vi "Create Process.vi"(8 "error in (no error)":errorcluster, 10 "Sequence":string[](array[string]), 11 "Process Model in":refnum<class "Process Model.lvclass">) -> (0 "error out":errorcluster, 3 "Process Model out":refnum<class "Process Model.lvclass">)   [LabVIEW 2017, in "Process Model.lvlib" / "Process Model.lvclass"]
uses:
  <vilib>/gpm_packages/@cs/Car wash/Process Model/Process Model/Process Model.lvclass
  <vilib>/gpm_packages/@cs/test-executive/Source/Test Executive/TestExecutive Ref/TestExecutive Ref.lvclass
  <vilib>/gpm_packages/@cs/test-executive/Source/Test Executive/TestExecutive/Test Executive.lvclass
  <vilib>/gpm_packages/@cs/Car wash/Process Model/Process Steps/Set Desired Station/Set Desired Station.lvclass
  <vilib>/gpm_packages/@cs/test-executive/Source/Test Executive/Executioner/Executioner.lvclass
  148baa78-ab47-4ac2-a908-5eab3e623dd9.vi
  2634eeb6-4d42-4bc9-82b5-37b6fa3864e8.vi
  <vilib>/gpm_packages/@cs/Car wash/Process Model/Process Steps/Start Under Body Wash/Start Under Body Wash.lvclass
  e4c6561f-6417-4e21-a938-d836dda1ae79.vi
  <vilib>/gpm_packages/@cs/Car wash/Process Model/Process Steps/Wait/Wait.lvclass
  c08b7c41-2827-4655-bbff-50a6a7c73d4f.vi
  <vilib>/gpm_packages/@cs/Car wash/Process Model/Process Steps/Stop Under Body Wash/Stop Under Body Wash.lvclass
  f4110d32-f2ed-440d-ac33-f75860a216d9.vi
  <vilib>/gpm_packages/@cs/Car wash/Process Model/Process Steps/Start Bug Remover/Start Bug Remover.lvclass
  38c94591-f339-49dc-907e-f278cc2e51ff.vi
  <vilib>/gpm_packages/@cs/Car wash/Process Model/Process Steps/Stop Bug Remover/Stop Bug Remover.lvclass
  f7fd6c87-c4ae-48d3-978c-34364638cacd.vi
  <vilib>/gpm_packages/@cs/Car wash/Process Model/Process Steps/Start Pre-Soak/Start Pre-Soak.lvclass
  975d0a21-73d7-4169-b5a5-a1460635b443.vi
  <vilib>/gpm_packages/@cs/Car wash/Process Model/Process Steps/Stop Pre-Soak/Stop Pre-Soak.lvclass
  07d419d3-c35c-4609-8eee-0d116beaf2ef.vi
  <vilib>/gpm_packages/@cs/Car wash/Process Model/Process Steps/Start High Pressure Wash/Start High Pressure Wash.lvclass
  43e1845e-1a9b-47c3-a4cd-faa5e21737b1.vi
  <vilib>/gpm_packages/@cs/Car wash/Process Model/Process Steps/Stop High Pressure Wash/Stop High Pressure Wash.lvclass
  178d77fd-57ed-4720-a89c-829f4238c359.vi
  <vilib>/gpm_packages/@cs/Car wash/Process Model/Process Steps/Start Low Pressure Wax/Start Low Pressure Wax.lvclass
  1292d9c1-c930-4c00-a311-9cd2a177a2f0.vi
  <vilib>/gpm_packages/@cs/Car wash/Process Model/Process Steps/Stop Low Pressure Wax/Stop Low Pressure Wax.lvclass
  f597536c-d9cd-43c5-8d13-b9a318907401.vi
  <vilib>/gpm_packages/@cs/Car wash/Process Model/Process Steps/Start Air Dry/Start Air Dry.lvclass
  adc60016-b060-4db0-b707-518d8c9f6844.vi
  <vilib>/gpm_packages/@cs/Car wash/Process Model/Process Steps/Stop Air Dry/Stop Air Dry.lvclass
  58db1882-6cd1-40bb-add2-e4b922ecf0a5.vi
  <vilib>/gpm_packages/@cs/Car wash/Process Model/Process Steps/Start Spot Free Rinse/Start Spot Free Rinse.lvclass
  7577cb98-fec7-4599-9fc4-8f1fe5d712e2.vi
  <vilib>/gpm_packages/@cs/Car wash/Process Model/Process Steps/Stop Spot Free Rinse/Stop Spot Free Rinse.lvclass
  fc6307b7-2fc7-402e-94d3-f9c0f8fc91bb.vi
  <vilib>/gpm_packages/@cs/Car wash/Process Model/Process Steps/Start Tire Shine Foam/Start Tire Shine Foam.lvclass
  13563156-251b-405d-92c3-91e0f6b0e34d.vi
  <vilib>/gpm_packages/@cs/Car wash/Process Model/Process Steps/Stop Tire Shine Foam/Stop Tire Shine Foam.lvclass
  640e79f8-33ad-472c-aa49-3045e868de91.vi
  <vilib>/gpm_packages/@cs/Car wash/Process Model/Process Steps/Exit/Exit.lvclass
  b05cf328-ca6c-4f2d-8483-90633d7417f2.vi
  <vilib>/gpm_packages/@cs/Car wash/Process Model/Process Steps/Initialize HMI/Initialize HMI.lvclass
  C:/Program Files/National Instruments/LabVIEW 2017/vi.lib/gpm_packages/@cs/test-executive/Source/Test Executive/ITestExecutive/ITest Executive.lvclass
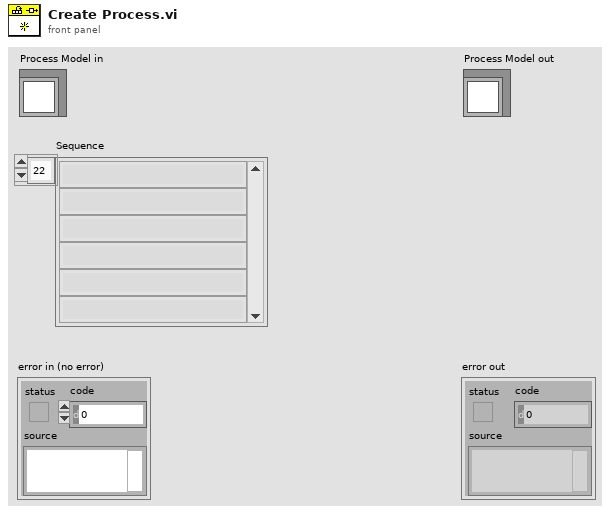
[diagram p1: front panel]
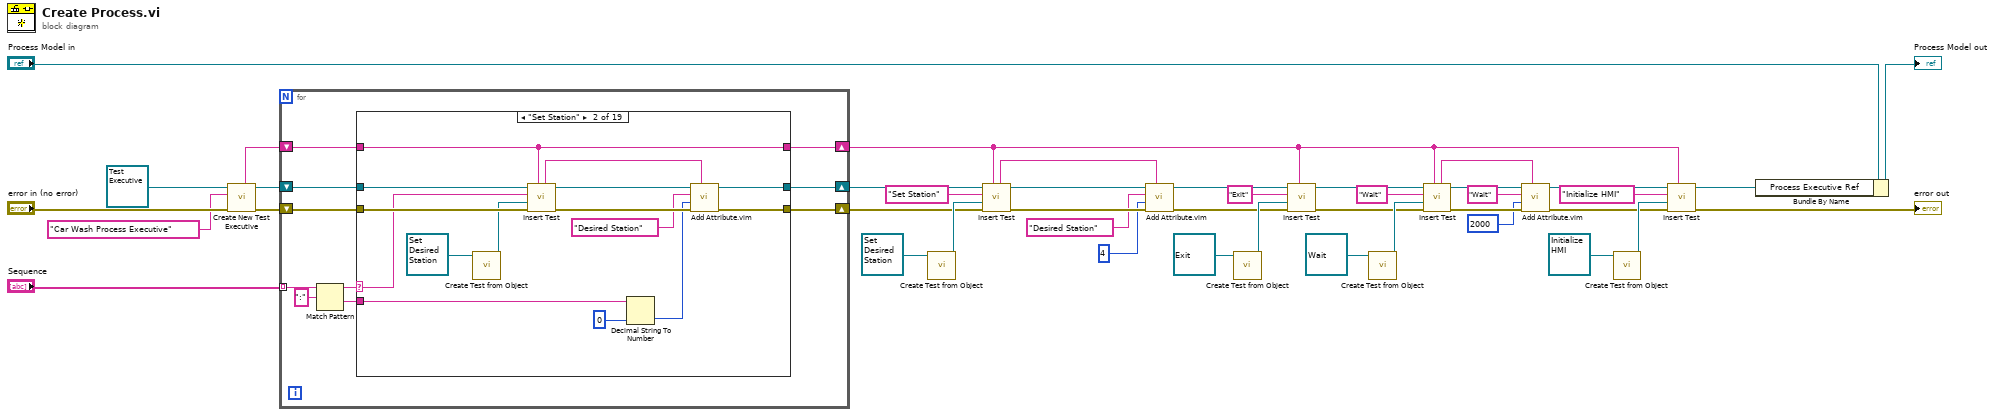
[diagram p0: block diagram]
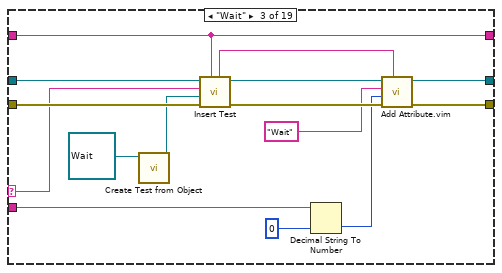
[diagram p3: hidden frame]
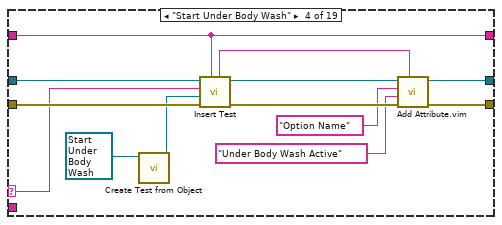
[diagram p4: hidden frame]
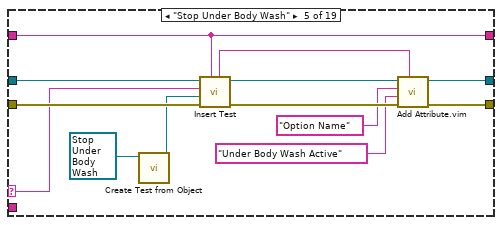
[diagram p5: hidden frame]
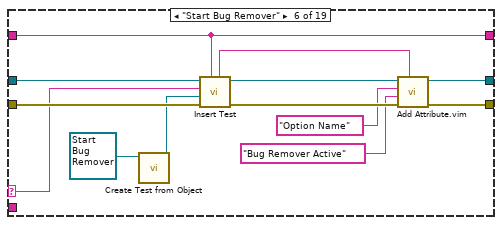
[diagram p6: hidden frame]
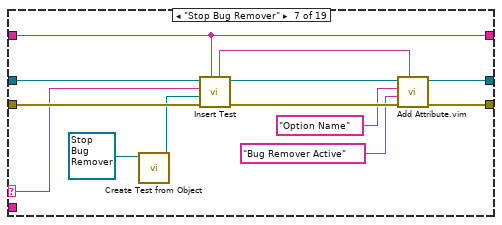
[diagram p7: hidden frame]
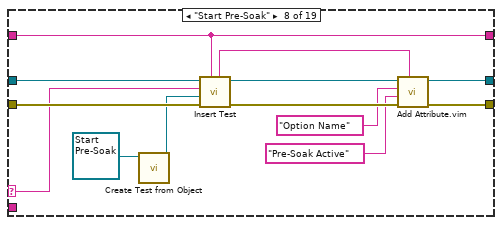
[diagram p8: hidden frame]
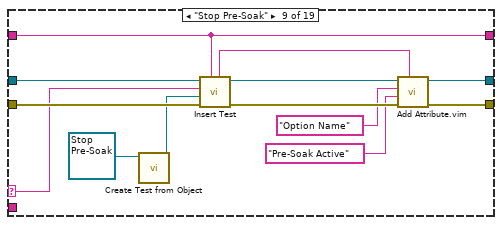
[diagram p9: hidden frame]
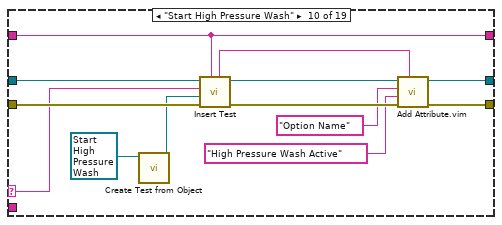
[diagram p10: hidden frame]
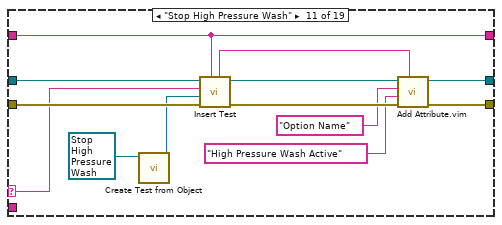
[diagram p11: hidden frame]
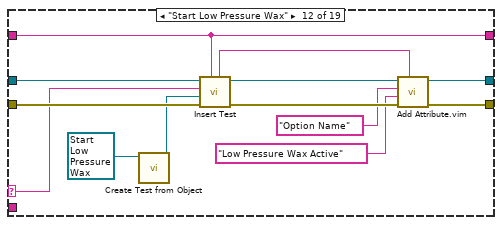
[diagram p12: hidden frame]
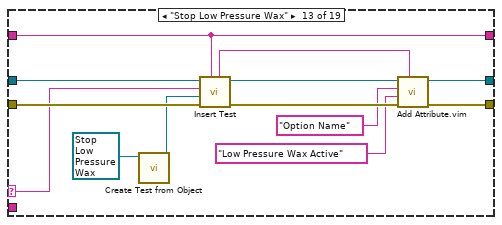
[diagram p13: hidden frame]
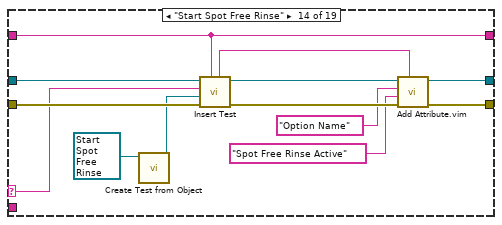
[diagram p14: hidden frame]
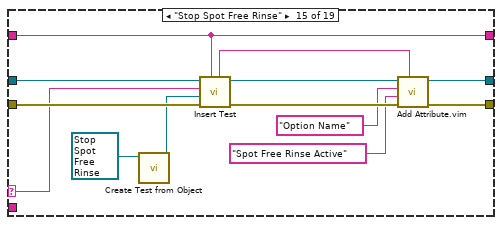
[diagram p15: hidden frame]
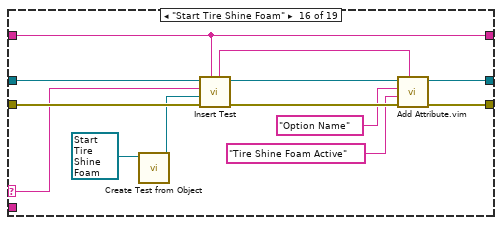
[diagram p16: hidden frame]
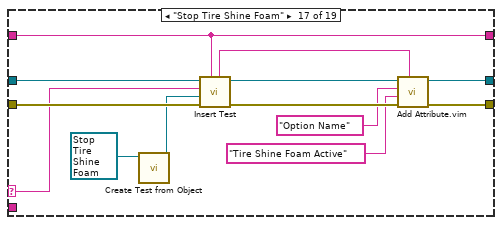
[diagram p17: hidden frame]
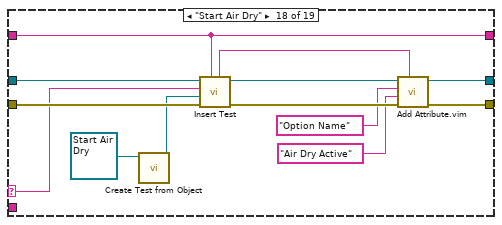
[diagram p18: hidden frame]
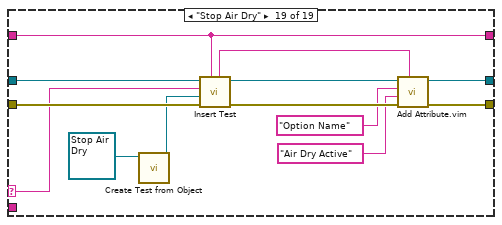
[diagram p19: hidden frame]
diagram:
  n1 = call <vilib>:"Create New Test Executive.vi"("error in (no error)"="error in (no error)", "Name"="Car Wash Process Executive", "Test Executive"=refnum<class "Test Executive.lvclass"> refnum ("Test Executive.lvlib:Test Executive.lvclass")) -> ("error out"=w36:errorcluster, "Test Executive Ref"=w37:refnum<data-value>, "Test Executive ID out"=w34:string)  [unwired: 6 in]
  n2 = for {
    shift-right: [w51] -> w27
    shift-left: w37 -> [w52]
    shift-right: [w49] -> w26
    shift-left: w36 -> [w50]
    tunnel: "Sequence" -> [w48] mode=indexing
    shift-right: [w43] -> w4
    shift-left: w34 -> [w44]
    n3 = Match Pattern(string=w48, regular expression=":") -> (before substring=w47:string, after substring=w46:string)  [unwired: 1 in, 2 out]
    n4 = case shown="\"Set Station\"" w47 {
      selector: w47 -> [_ w68 w82 w95 w108 w121 w134 w147 w160 w173 w186 w199 w212 w225 w238 w251 w264 w277 w290]
      tunnel: w52 -> [w55 w70 w85 w98 w111 w124 w137 w150 w163 w176 w189 w202 w215 w228 w241 w254 w267 w280 w293]
      tunnel: [w55 w64 w79 w92 w105 w118 w131 w144 w157 w170 w183 w196 w209 w222 w235 w248 w261 w274 w287] -> w51
      tunnel: w50 -> [w54 w69 w84 w97 w110 w123 w136 w149 w162 w175 w188 w201 w214 w227 w240 w253 w266 w279 w292]
      tunnel: [w54 w62 w77 w90 w103 w116 w129 w142 w155 w168 w181 w194 w207 w220 w233 w246 w259 w272 w285] -> w49
      tunnel: w46 -> [_ w59 w75 _ _ _ _ _ _ _ _ _ _ _ _ _ _ _ _]
      tunnel: w44 -> [w53 w56 w83 w96 w109 w122 w135 w148 w161 w174 w187 w200 w213 w226 w239 w252 w265 w278 w291]
      tunnel: [w53 w56 w83 w96 w109 w122 w135 w148 w161 w174 w187 w200 w213 w226 w239 w252 w265 w278 w291] -> w43
      frame Default {
      }
      frame "Set Station" {
        n5 = call <vilib>:"Create Test from Object.vi"("Test"=refnum<class "Set Desired Station.lvclass"> refnum ("Set Desired Station.lvclass")) -> ("Test"=w66:refnum<class "Executioner.lvclass">)  [unwired: 10 in]
        n6 = call <vilib>:"Insert Test.vi"("Parent ID"=w56, "error in (no error)"=w69, "Test"=w66, "Name"=w68, "Test Executive Ref"=w70) -> ("error out"=w63:errorcluster, "Test Executive Ref out"=w65:refnum<data-value>, "Unique ID out"=w61:string)  [unwired: 3 in, 1 out]
        n7 = Decimal String To Number(string=w59, default (0L)=u8 0) -> (number=w57:u8)  [unwired: 1 in, 1 out]
        n8 = call "Add Attribute.vim"("ID"=w61, "error in (no error)"=w63, "Attribute"=w57, "Attribute Name"="Desired Station" ("Item Name"), "Test Executive Ref"=w65) -> ("error out"=w62:errorcluster, "Test Executive Ref out"=w64:refnum<data-value>)  [unwired: 3 in, 2 out]
      }
      frame "Wait" {
        n9 = call <vilib>:"Create Test from Object.vi"("Test"=refnum<class "Wait.lvclass"> refnum ("Wait.lvclass")) -> ("Test"=w81:refnum<class "Executioner.lvclass">)  [unwired: 10 in]
        n10 = call <vilib>:"Insert Test.vi"("Parent ID"=w83, "error in (no error)"=w84, "Test"=w81, "Name"=w82, "Test Executive Ref"=w85) -> ("error out"=w78:errorcluster, "Test Executive Ref out"=w80:refnum<data-value>, "Unique ID out"=w76:string)  [unwired: 3 in, 1 out]
        n11 = Decimal String To Number(string=w75, default (0L)=0) -> (number=w74:i32)  [unwired: 1 in, 1 out]
        n12 = call "Add Attribute.vim"("ID"=w76, "error in (no error)"=w78, "Attribute"=w74, "Attribute Name"="Wait" ("Item Name"), "Test Executive Ref"=w80) -> ("error out"=w77:errorcluster, "Test Executive Ref out"=w79:refnum<data-value>)  [unwired: 3 in, 2 out]
      }
      frame "Start Under Body Wash" {
        n13 = call <vilib>:"Create Test from Object.vi"("Test"=refnum<class "Start Under Body Wash.lvclass"> refnum ("Start Under Body Wash.lvclass")) -> ("Test"=w94:refnum<class "Executioner.lvclass">)  [unwired: 10 in]
        n14 = call <vilib>:"Insert Test.vi"("Parent ID"=w96, "error in (no error)"=w97, "Test"=w94, "Name"=w95, "Test Executive Ref"=w98) -> ("error out"=w91:errorcluster, "Test Executive Ref out"=w93:refnum<data-value>, "Unique ID out"=w89:string)  [unwired: 3 in, 1 out]
        n15 = call "Add Attribute.vim"("ID"=w89, "error in (no error)"=w91, "Attribute"="Under Body Wash Active" ("Item Name"), "Attribute Name"="Option Name" ("Item Name"), "Test Executive Ref"=w93) -> ("error out"=w90:errorcluster, "Test Executive Ref out"=w92:refnum<data-value>)  [unwired: 3 in, 2 out]
      }
      frame "Stop Under Body Wash" {
        n16 = call <vilib>:"Create Test from Object.vi"("Test"=refnum<class "Stop Under Body Wash.lvclass"> refnum ("Stop Under Body Wash.lvclass")) -> ("Test"=w107:refnum<class "Executioner.lvclass">)  [unwired: 10 in]
        n17 = call <vilib>:"Insert Test.vi"("Parent ID"=w109, "error in (no error)"=w110, "Test"=w107, "Name"=w108, "Test Executive Ref"=w111) -> ("error out"=w104:errorcluster, "Test Executive Ref out"=w106:refnum<data-value>, "Unique ID out"=w102:string)  [unwired: 3 in, 1 out]
        n18 = call "Add Attribute.vim"("ID"=w102, "error in (no error)"=w104, "Attribute"="Under Body Wash Active" ("Item Name"), "Attribute Name"="Option Name" ("Item Name"), "Test Executive Ref"=w106) -> ("error out"=w103:errorcluster, "Test Executive Ref out"=w105:refnum<data-value>)  [unwired: 3 in, 2 out]
      }
      frame "Start Bug Remover" {
        n19 = call <vilib>:"Create Test from Object.vi"("Test"=refnum<class "Start Bug Remover.lvclass"> refnum ("Start Bug Remover.lvclass")) -> ("Test"=w120:refnum<class "Executioner.lvclass">)  [unwired: 10 in]
        n20 = call <vilib>:"Insert Test.vi"("Parent ID"=w122, "error in (no error)"=w123, "Test"=w120, "Name"=w121, "Test Executive Ref"=w124) -> ("error out"=w117:errorcluster, "Test Executive Ref out"=w119:refnum<data-value>, "Unique ID out"=w115:string)  [unwired: 3 in, 1 out]
        n21 = call "Add Attribute.vim"("ID"=w115, "error in (no error)"=w117, "Attribute"="Bug Remover Active" ("Item Name"), "Attribute Name"="Option Name" ("Item Name"), "Test Executive Ref"=w119) -> ("error out"=w116:errorcluster, "Test Executive Ref out"=w118:refnum<data-value>)  [unwired: 3 in, 2 out]
      }
      frame "Stop Bug Remover" {
        n22 = call <vilib>:"Create Test from Object.vi"("Test"=refnum<class "Stop Bug Remover.lvclass"> refnum ("Stop Bug Remover.lvclass")) -> ("Test"=w133:refnum<class "Executioner.lvclass">)  [unwired: 10 in]
        n23 = call <vilib>:"Insert Test.vi"("Parent ID"=w135, "error in (no error)"=w136, "Test"=w133, "Name"=w134, "Test Executive Ref"=w137) -> ("error out"=w130:errorcluster, "Test Executive Ref out"=w132:refnum<data-value>, "Unique ID out"=w128:string)  [unwired: 3 in, 1 out]
        n24 = call "Add Attribute.vim"("ID"=w128, "error in (no error)"=w130, "Attribute"="Bug Remover Active" ("Item Name"), "Attribute Name"="Option Name" ("Item Name"), "Test Executive Ref"=w132) -> ("error out"=w129:errorcluster, "Test Executive Ref out"=w131:refnum<data-value>)  [unwired: 3 in, 2 out]
      }
      frame "Start Pre-Soak" {
        n25 = call <vilib>:"Create Test from Object.vi"("Test"=refnum<class "Start Pre-Soak.lvclass"> refnum ("Start Pre-Soak.lvclass")) -> ("Test"=w146:refnum<class "Executioner.lvclass">)  [unwired: 10 in]
        n26 = call <vilib>:"Insert Test.vi"("Parent ID"=w148, "error in (no error)"=w149, "Test"=w146, "Name"=w147, "Test Executive Ref"=w150) -> ("error out"=w143:errorcluster, "Test Executive Ref out"=w145:refnum<data-value>, "Unique ID out"=w141:string)  [unwired: 3 in, 1 out]
        n27 = call "Add Attribute.vim"("ID"=w141, "error in (no error)"=w143, "Attribute"="Pre-Soak Active" ("Item Name"), "Attribute Name"="Option Name" ("Item Name"), "Test Executive Ref"=w145) -> ("error out"=w142:errorcluster, "Test Executive Ref out"=w144:refnum<data-value>)  [unwired: 3 in, 2 out]
      }
      frame "Stop Pre-Soak" {
        n28 = call <vilib>:"Create Test from Object.vi"("Test"=refnum<class "Stop Pre-Soak.lvclass"> refnum ("Stop Pre-Soak.lvclass")) -> ("Test"=w159:refnum<class "Executioner.lvclass">)  [unwired: 10 in]
        n29 = call <vilib>:"Insert Test.vi"("Parent ID"=w161, "error in (no error)"=w162, "Test"=w159, "Name"=w160, "Test Executive Ref"=w163) -> ("error out"=w156:errorcluster, "Test Executive Ref out"=w158:refnum<data-value>, "Unique ID out"=w154:string)  [unwired: 3 in, 1 out]
        n30 = call "Add Attribute.vim"("ID"=w154, "error in (no error)"=w156, "Attribute"="Pre-Soak Active" ("Item Name"), "Attribute Name"="Option Name" ("Item Name"), "Test Executive Ref"=w158) -> ("error out"=w155:errorcluster, "Test Executive Ref out"=w157:refnum<data-value>)  [unwired: 3 in, 2 out]
      }
      frame "Start High Pressure Wash" {
        n31 = call <vilib>:"Create Test from Object.vi"("Test"=refnum<class "Start High Pressure Wash.lvclass"> refnum ("Start High Pressure Wash.lvclass")) -> ("Test"=w172:refnum<class "Executioner.lvclass">)  [unwired: 10 in]
        n32 = call <vilib>:"Insert Test.vi"("Parent ID"=w174, "error in (no error)"=w175, "Test"=w172, "Name"=w173, "Test Executive Ref"=w176) -> ("error out"=w169:errorcluster, "Test Executive Ref out"=w171:refnum<data-value>, "Unique ID out"=w167:string)  [unwired: 3 in, 1 out]
        n33 = call "Add Attribute.vim"("ID"=w167, "error in (no error)"=w169, "Attribute"="High Pressure Wash Active" ("Item Name"), "Attribute Name"="Option Name" ("Item Name"), "Test Executive Ref"=w171) -> ("error out"=w168:errorcluster, "Test Executive Ref out"=w170:refnum<data-value>)  [unwired: 3 in, 2 out]
      }
      frame "Stop High Pressure Wash" {
        n34 = call <vilib>:"Create Test from Object.vi"("Test"=refnum<class "Stop High Pressure Wash.lvclass"> refnum ("Stop High Pressure Wash.lvclass")) -> ("Test"=w185:refnum<class "Executioner.lvclass">)  [unwired: 10 in]
        n35 = call <vilib>:"Insert Test.vi"("Parent ID"=w187, "error in (no error)"=w188, "Test"=w185, "Name"=w186, "Test Executive Ref"=w189) -> ("error out"=w182:errorcluster, "Test Executive Ref out"=w184:refnum<data-value>, "Unique ID out"=w180:string)  [unwired: 3 in, 1 out]
        n36 = call "Add Attribute.vim"("ID"=w180, "error in (no error)"=w182, "Attribute"="High Pressure Wash Active" ("Item Name"), "Attribute Name"="Option Name" ("Item Name"), "Test Executive Ref"=w184) -> ("error out"=w181:errorcluster, "Test Executive Ref out"=w183:refnum<data-value>)  [unwired: 3 in, 2 out]
      }
      frame "Start Low Pressure Wax" {
        n37 = call <vilib>:"Create Test from Object.vi"("Test"=refnum<class "Start Low Pressure Wax.lvclass"> refnum ("Start Low Pressure Wax.lvclass")) -> ("Test"=w198:refnum<class "Executioner.lvclass">)  [unwired: 10 in]
        n38 = call <vilib>:"Insert Test.vi"("Parent ID"=w200, "error in (no error)"=w201, "Test"=w198, "Name"=w199, "Test Executive Ref"=w202) -> ("error out"=w195:errorcluster, "Test Executive Ref out"=w197:refnum<data-value>, "Unique ID out"=w193:string)  [unwired: 3 in, 1 out]
        n39 = call "Add Attribute.vim"("ID"=w193, "error in (no error)"=w195, "Attribute"="Low Pressure Wax Active" ("Item Name"), "Attribute Name"="Option Name" ("Item Name"), "Test Executive Ref"=w197) -> ("error out"=w194:errorcluster, "Test Executive Ref out"=w196:refnum<data-value>)  [unwired: 3 in, 2 out]
      }
      frame "Stop Low Pressure Wax" {
        n40 = call <vilib>:"Create Test from Object.vi"("Test"=refnum<class "Stop Low Pressure Wax.lvclass"> refnum ("Stop Low Pressure Wax.lvclass")) -> ("Test"=w211:refnum<class "Executioner.lvclass">)  [unwired: 10 in]
        n41 = call <vilib>:"Insert Test.vi"("Parent ID"=w213, "error in (no error)"=w214, "Test"=w211, "Name"=w212, "Test Executive Ref"=w215) -> ("error out"=w208:errorcluster, "Test Executive Ref out"=w210:refnum<data-value>, "Unique ID out"=w206:string)  [unwired: 3 in, 1 out]
        n42 = call "Add Attribute.vim"("ID"=w206, "error in (no error)"=w208, "Attribute"="Low Pressure Wax Active" ("Item Name"), "Attribute Name"="Option Name" ("Item Name"), "Test Executive Ref"=w210) -> ("error out"=w207:errorcluster, "Test Executive Ref out"=w209:refnum<data-value>)  [unwired: 3 in, 2 out]
      }
      frame "Start Spot Free Rinse" {
        n43 = call <vilib>:"Create Test from Object.vi"("Test"=refnum<class "Start Spot Free Rinse.lvclass"> refnum ("Start Spot Free Rinse.lvclass")) -> ("Test"=w224:refnum<class "Executioner.lvclass">)  [unwired: 10 in]
        n44 = call <vilib>:"Insert Test.vi"("Parent ID"=w226, "error in (no error)"=w227, "Test"=w224, "Name"=w225, "Test Executive Ref"=w228) -> ("error out"=w221:errorcluster, "Test Executive Ref out"=w223:refnum<data-value>, "Unique ID out"=w219:string)  [unwired: 3 in, 1 out]
        n45 = call "Add Attribute.vim"("ID"=w219, "error in (no error)"=w221, "Attribute"="Spot Free Rinse Active" ("Item Name"), "Attribute Name"="Option Name" ("Item Name"), "Test Executive Ref"=w223) -> ("error out"=w220:errorcluster, "Test Executive Ref out"=w222:refnum<data-value>)  [unwired: 3 in, 2 out]
      }
      frame "Stop Spot Free Rinse" {
        n46 = call <vilib>:"Create Test from Object.vi"("Test"=refnum<class "Stop Spot Free Rinse.lvclass"> refnum ("Stop Spot Free Rinse.lvclass")) -> ("Test"=w237:refnum<class "Executioner.lvclass">)  [unwired: 10 in]
        n47 = call <vilib>:"Insert Test.vi"("Parent ID"=w239, "error in (no error)"=w240, "Test"=w237, "Name"=w238, "Test Executive Ref"=w241) -> ("error out"=w234:errorcluster, "Test Executive Ref out"=w236:refnum<data-value>, "Unique ID out"=w232:string)  [unwired: 3 in, 1 out]
        n48 = call "Add Attribute.vim"("ID"=w232, "error in (no error)"=w234, "Attribute"="Spot Free Rinse Active" ("Item Name"), "Attribute Name"="Option Name" ("Item Name"), "Test Executive Ref"=w236) -> ("error out"=w233:errorcluster, "Test Executive Ref out"=w235:refnum<data-value>)  [unwired: 3 in, 2 out]
      }
      frame "Start Tire Shine Foam" {
        n49 = call <vilib>:"Create Test from Object.vi"("Test"=refnum<class "Start Tire Shine Foam.lvclass"> refnum ("Start Tire Shine Foam.lvclass")) -> ("Test"=w250:refnum<class "Executioner.lvclass">)  [unwired: 10 in]
        n50 = call <vilib>:"Insert Test.vi"("Parent ID"=w252, "error in (no error)"=w253, "Test"=w250, "Name"=w251, "Test Executive Ref"=w254) -> ("error out"=w247:errorcluster, "Test Executive Ref out"=w249:refnum<data-value>, "Unique ID out"=w245:string)  [unwired: 3 in, 1 out]
        n51 = call "Add Attribute.vim"("ID"=w245, "error in (no error)"=w247, "Attribute"="Tire Shine Foam Active" ("Item Name"), "Attribute Name"="Option Name" ("Item Name"), "Test Executive Ref"=w249) -> ("error out"=w246:errorcluster, "Test Executive Ref out"=w248:refnum<data-value>)  [unwired: 3 in, 2 out]
      }
      frame "Stop Tire Shine Foam" {
        n52 = call <vilib>:"Create Test from Object.vi"("Test"=refnum<class "Stop Tire Shine Foam.lvclass"> refnum ("Stop Tire Shine Foam.lvclass")) -> ("Test"=w263:refnum<class "Executioner.lvclass">)  [unwired: 10 in]
        n53 = call <vilib>:"Insert Test.vi"("Parent ID"=w265, "error in (no error)"=w266, "Test"=w263, "Name"=w264, "Test Executive Ref"=w267) -> ("error out"=w260:errorcluster, "Test Executive Ref out"=w262:refnum<data-value>, "Unique ID out"=w258:string)  [unwired: 3 in, 1 out]
        n54 = call "Add Attribute.vim"("ID"=w258, "error in (no error)"=w260, "Attribute"="Tire Shine Foam Active" ("Item Name"), "Attribute Name"="Option Name" ("Item Name"), "Test Executive Ref"=w262) -> ("error out"=w259:errorcluster, "Test Executive Ref out"=w261:refnum<data-value>)  [unwired: 3 in, 2 out]
      }
      frame "Start Air Dry" {
        n55 = call <vilib>:"Create Test from Object.vi"("Test"=refnum<class "Start Air Dry.lvclass"> refnum ("Start Air Dry.lvclass")) -> ("Test"=w276:refnum<class "Executioner.lvclass">)  [unwired: 10 in]
        n56 = call <vilib>:"Insert Test.vi"("Parent ID"=w278, "error in (no error)"=w279, "Test"=w276, "Name"=w277, "Test Executive Ref"=w280) -> ("error out"=w273:errorcluster, "Test Executive Ref out"=w275:refnum<data-value>, "Unique ID out"=w271:string)  [unwired: 3 in, 1 out]
        n57 = call "Add Attribute.vim"("ID"=w271, "error in (no error)"=w273, "Attribute"="Air Dry Active" ("Item Name"), "Attribute Name"="Option Name" ("Item Name"), "Test Executive Ref"=w275) -> ("error out"=w272:errorcluster, "Test Executive Ref out"=w274:refnum<data-value>)  [unwired: 3 in, 2 out]
      }
      frame "Stop Air Dry" {
        n58 = call <vilib>:"Create Test from Object.vi"("Test"=refnum<class "Stop Air Dry.lvclass"> refnum ("Stop Air Dry.lvclass")) -> ("Test"=w289:refnum<class "Executioner.lvclass">)  [unwired: 10 in]
        n59 = call <vilib>:"Insert Test.vi"("Parent ID"=w291, "error in (no error)"=w292, "Test"=w289, "Name"=w290, "Test Executive Ref"=w293) -> ("error out"=w286:errorcluster, "Test Executive Ref out"=w288:refnum<data-value>, "Unique ID out"=w284:string)  [unwired: 3 in, 1 out]
        n60 = call "Add Attribute.vim"("ID"=w284, "error in (no error)"=w286, "Attribute"="Air Dry Active" ("Item Name"), "Attribute Name"="Option Name" ("Item Name"), "Test Executive Ref"=w288) -> ("error out"=w285:errorcluster, "Test Executive Ref out"=w287:refnum<data-value>)  [unwired: 3 in, 2 out]
      }
    }
  }
  n61 = call <vilib>:"Create Test from Object.vi"("Test"=refnum<class "Set Desired Station.lvclass"> refnum ("Set Desired Station.lvclass")) -> ("Test"=w32:refnum<class "Executioner.lvclass">)  [unwired: 10 in]
  n62 = call <vilib>:"Insert Test.vi"("Parent ID"=w4, "error in (no error)"=w26, "Test"=w32, "Name"="Set Station", "Test Executive Ref"=w27) -> ("error out"=w30:errorcluster, "Test Executive Ref out"=w31:refnum<data-value>, "Unique ID out"=w29:string)  [unwired: 3 in, 1 out]
  n63 = call "Add Attribute.vim"("ID"=w29, "error in (no error)"=w30, "Attribute"=u8 4, "Attribute Name"="Desired Station" ("Item Name"), "Test Executive Ref"=w31) -> ("error out"=w20:errorcluster, "Test Executive Ref out"=w21:refnum<data-value>)  [unwired: 3 in, 2 out]
  n64 = call <vilib>:"Create Test from Object.vi"("Test"=refnum<class "Exit.lvclass"> refnum ("Exit.lvclass")) -> ("Test"=w22:refnum<class "Executioner.lvclass">)  [unwired: 10 in]
  n65 = call <vilib>:"Insert Test.vi"("Parent ID"=w4, "error in (no error)"=w20, "Test"=w22, "Name"="Exit", "Test Executive Ref"=w21) -> ("error out"=w11:errorcluster, "Test Executive Ref out"=w12:refnum<data-value>)  [unwired: 3 in, 2 out]
  n66 = call <vilib>:"Create Test from Object.vi"("Test"=refnum<class "Wait.lvclass"> refnum ("Wait.lvclass")) -> ("Test"=w18:refnum<class "Executioner.lvclass">)  [unwired: 10 in]
  n67 = call <vilib>:"Insert Test.vi"("Parent ID"=w4, "error in (no error)"=w11, "Test"=w18, "Name"="Wait", "Test Executive Ref"=w12) -> ("error out"=w16:errorcluster, "Test Executive Ref out"=w17:refnum<data-value>, "Unique ID out"=w15:string)  [unwired: 3 in, 1 out]
  n68 = call "Add Attribute.vim"("ID"=w15, "error in (no error)"=w16, "Attribute"=2000, "Attribute Name"="Wait" ("Item Name"), "Test Executive Ref"=w17) -> ("error out"=w6:errorcluster, "Test Executive Ref out"=w8:refnum<data-value>)  [unwired: 3 in, 2 out]
  n69 = call <vilib>:"Create Test from Object.vi"("Test"=refnum<class "Initialize HMI.lvclass"> refnum ("Initialize HMI.lvclass")) -> ("Test"=w9:refnum<class "Executioner.lvclass">)  [unwired: 10 in]
  n70 = call <vilib>:"Insert Test.vi"("Parent ID"=w4, "error in (no error)"=w6, "Test"=w9, "Name"="Initialize HMI", "Test Executive Ref"=w8) -> ("error out"=→"error out":errorcluster, "Test Executive Ref out"=w7:refnum<data-value>)  [unwired: 3 in, 2 out]
  n71 = Bundle By Name(cluster="Process Model in", "Process Executive Ref"=w7) -> (→"Process Model out":refnum<class "Process Model.lvclass">)
